vi "Configure Steps.vi"(8 "error in (no error)":errorcluster, 11 "Test Measurement in":refnum<class "Test Measurement.lvclass">) -> (0 "error out":errorcluster, 3 "Test Measurement out":refnum<class "Test Measurement.lvclass">)   [LabVIEW 2016, in "Test Measurement.lvclass"]
uses:
  Test Measurement.lvclass
  Plugins/QPA Measurement.lvlibp/QPA Measurement.lvclass
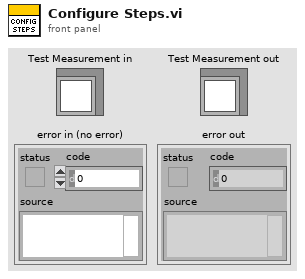
[diagram p1: front panel]
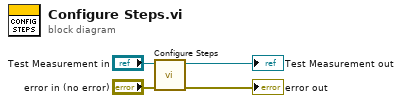
[diagram p0: block diagram]
diagram:
  n1 = call-parent "Configure Steps.vi"("error in (no error)"="error in (no error)", "QPA Measurement in"="Test Measurement in") -> ("error out"=→"error out":errorcluster, "QPA Measurement out"=→"Test Measurement out":refnum<class "Test Measurement.lvclass">)  [unwired: 8 in]
